vi "Update Position Array.vi"(9 "position":dbl, 10 "Axis":i32, 11 "Positions in":dbl[](array[numeric])) -> (3 "Positions out":dbl[](array[numeric]))   [LabVIEW 2019, in "ESP301.lvlib"]
uses:
  ESP301.lvlib
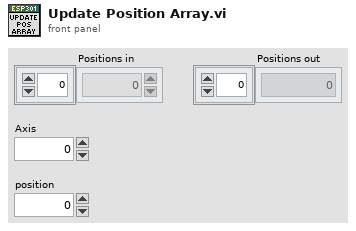
[diagram p1: front panel]
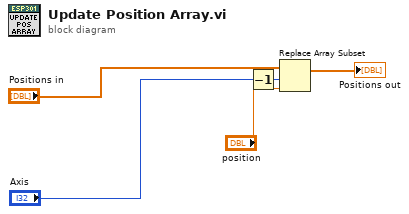
[diagram p0: block diagram]
diagram:
  n1 = Decrement(x="Axis") -> (x-1=w3:i32)
  n2 = Replace Array Subset(array="Positions in", new element="position", index=w3) -> (→"Positions out":dbl[])
